vi "Is Node Channel.vi"(8 "error in (no error)":errorcluster, 10 "Node Path":string, 11 "SDF Ref":refnum<k24>) -> (0 "error out":errorcluster, 2 "Is Channel?":bool)   [LabVIEW 2016, in "System Mapping Tool.lvlib"]
uses:
  System Mapping Tool.lvlib
  NationalInstruments.VeriStand.SystemDefinitionAPI
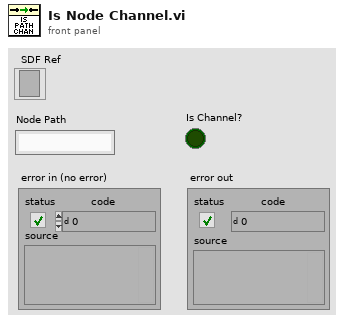
[diagram p1: front panel]
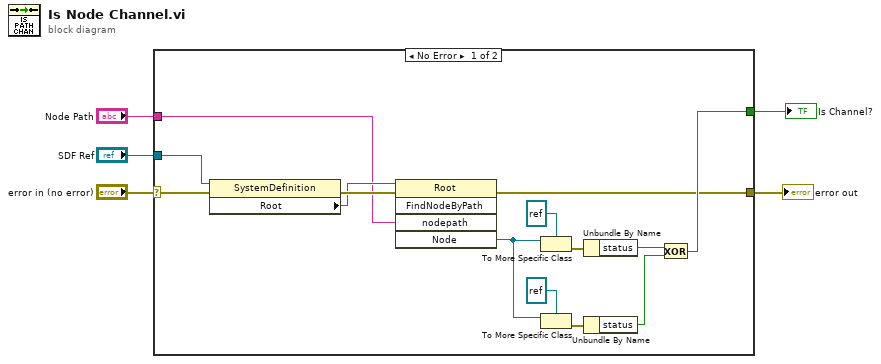
[diagram p0: block diagram]
diagram:
  n1 = case shown="No Error" "error in (no error)" {
    selector: "error in (no error)" -> [w19 w20]
    tunnel: [w6 w20] -> w4
    tunnel: "Node Path" -> [w16 _]
    tunnel: [w7 _] -> w2
    tunnel: "SDF Ref" -> [w15 _]
    frame No Error {
      n2 = property class="SystemDefinition"(reference=w15, error in=w19) -> (error out=w18:errorcluster, "Root"=w17:refnum<k24>)  [unwired: 1 out]
      n3 = invoke class="Root" method="FindNodeByPath"(reference=w17, error in=w18, "nodepath"=w16) -> (error out=w6:errorcluster, "Node"=w10:refnum<k24>)  [unwired: 2 in, 3 out]
      n4 = To More Specific Class(target class=refnum<k24> refnum ("new reference"), reference=w10) -> (error out=w12:errorcluster)  [unwired: 1 in, 1 out]
      n5 = To More Specific Class(target class=refnum<k24> refnum ("new reference"), reference=w10) -> (error out=w11:errorcluster)  [unwired: 1 in, 1 out]
      n6 = Unbundle By Name(w12) -> ("status"=w9:bool)
      n7 = Unbundle By Name(w11) -> ("status"=w8:bool)
      n8 = Exclusive Or(1:w8, 2:w9) -> (0:w7:bool)
    }
    frame Error {
    }
  }
  "error out" <- w4
  "Is Channel?" <- w2
